vi "check Cyclone Execution Status.vi"(8 "error in":errorcluster, 11 "cycloneHandle":u32) -> (0 "error out":errorcluster, 3 "function return":u32)   [LabVIEW 2021, in "CycloneControlSDK.lvlib"]
doc: "extern \"C\" uint32_t _cdecl checkCycloneExecutionStatus(uint32_t cycloneHandle);"
uses:
  CycloneControlSDK.lvlib
  CycloneControlSDK_64.dll
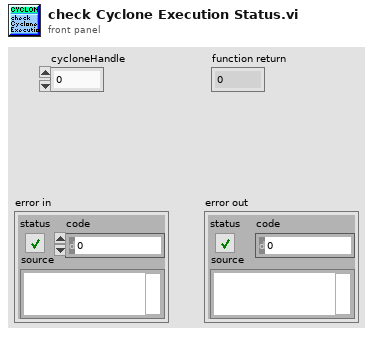
[diagram p1: front panel]
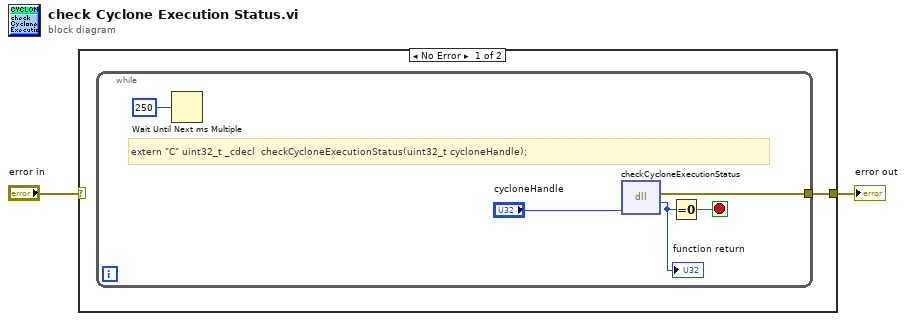
[diagram p0: block diagram]
diagram:
  n1 = case shown="No Error" "error in" {
    selector: "error in" -> [_ w9]
    tunnel: [w3 w9] -> w1
    frame No Error {
      n2 = while {
        tunnel: [w4] -> w3
        stop <- w6 stop-if-true
        # "extern \"C\" uint32_t _cdecl  checkCycloneExecutionStatus(uint32_t cycloneHandle);"
        n3 = Wait Until Next ms Multiple(millisecond multiple=u32 250) -> ()  [unwired: 1 out]
        n4 = dll-call lib="C:/PEMicro/cyclone/cycloneControl/controlsdk/examples/labview2018/user.lib/CycloneControlSDK/CycloneControlSDK_64.dll" fn="checkCycloneExecutionStatus"("cycloneHandle"="cycloneHandle") -> (error out=w4:errorcluster, "return type"=w5:u32)  [unwired: 4 in, 1 out]
        "function return" <- w5
        n5 = Equal To 0?(x=w5) -> (x = 0?=w6:bool)
      }
    }
    frame Error {
    }
  }
  "error out" <- w1
